vi "File Transfer From a Storage Device.vi"(7 "File Name ()":string, 8 "error in (no error)":errorcluster, 11 "VISA resource name":refnum<visa-resource-name>) -> (0 "error out":errorcluster, 2 "Data Block ()":string, 3 "VISA resource name out":refnum<visa-resource-name>)   [LabVIEW 2022 SP3, in "Agilent ENA Series.lvlib"]
doc: "Reads data from a file on the built-in storage device of the E5070B/E5071B/E5071C.\n\nBy reading out data with this VI and writing it to a file on the external controller, file transfer from the E5070B/E5071B/E5071C to the external controller can be realized. On the other hand, by reading out data from the external controller and writing it to a file on the E5070B/E5071B/E5071C with this function, file transfer from the external controller to the E5070B/E5071B/E5071C can be realized.\n\nSpecify the file name with the extension. If you want to specify \na file on the floppy disk\ndrive, you need to add \"A:\" at the beginning of the file name. When you use directory names and file name, separate them with \"/\" (slash) or \"\\\" (backslash)."
uses:
  <instrlib>/Agilent ENA Series/Agilent ENA Series.lvlib
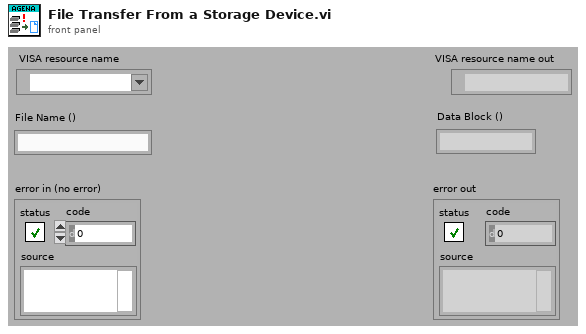
[diagram p1: front panel]
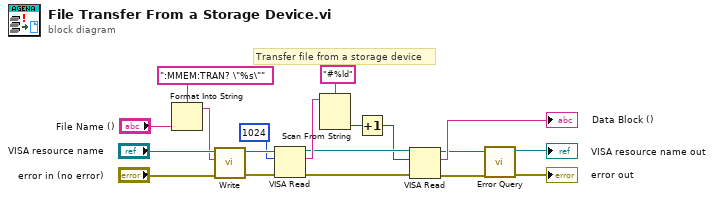
[diagram p0: block diagram]
diagram:
  # "Transfer file from a storage device"
  n1 = Format Into String(format string=":MMEM:TRAN? \"%s\"", "File Name ()") -> (resulting string=w15:string)  [unwired: 2 in, 1 out]
  n2 = call <instrlib>:"Write.vi"("error in (no error)"="error in (no error)", "String ()"=w15, "VISA resource name"="VISA resource name") -> ("error out"=w12:errorcluster, "VISA resource name out"=w13:refnum<visa-resource-name>)  [unwired: 6 in, 1 out]
  n3 = VISA Read(VISA resource name=w13, byte count=u32 1024, error in (no error)=w12) -> (VISA resource name out=w8:refnum<visa-resource-name>, read buffer=w9:string, error out=w7:errorcluster)  [unwired: 1 out]
  n4 = Scan From String(format string="#%ld", input string=w9) -> (output 1=w6:i32)  [unwired: 3 in, 3 out]
  n5 = Increment(x=w6) -> (x+1=w5:i32)
  n6 = VISA Read(VISA resource name=w8, byte count=w5, error in (no error)=w7) -> (VISA resource name out=w4:refnum<visa-resource-name>, read buffer=→"Data Block ()":string, error out=w3:errorcluster)  [unwired: 1 out]
  n7 = call <instrlib>:"Error Query.vi"("error in (no error)"=w3, "VISA resource name"=w4) -> ("error out"=→"error out":errorcluster, "VISA resource name out"=→"VISA resource name out":refnum<visa-resource-name>)  [unwired: 6 in, 2 out]
